vi "yaqc_home.vi"(8 "error in (no error)":errorcluster, 9 "Yaqc Client In":refnum<k38>, 10 "Python Module Path In":path, 11 "Python Session In":refnum<k35>) -> (0 "error out":errorcluster, 1 "Yaqc Client Out":refnum<k38>, 2 "Python Module Path Out":path, 3 "Python Session Out":refnum<k35>)   [LabVIEW 2022 SP3]
doc: "Initiates the homing procedure. The daemon will report as busy during the homing procedure. After the homing procedure is complete, the daemon will return to the current destination."
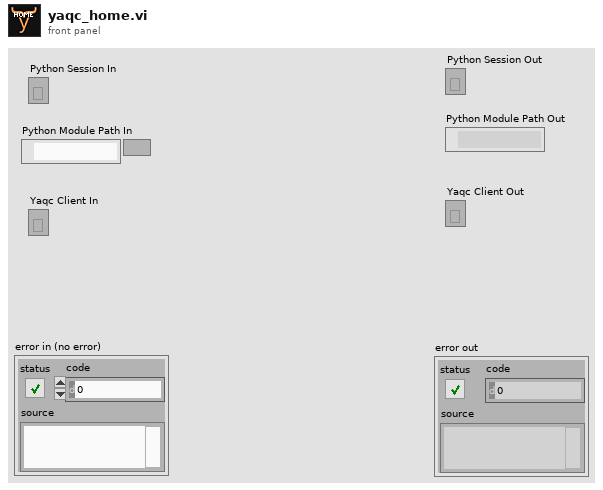
[diagram p1: front panel]
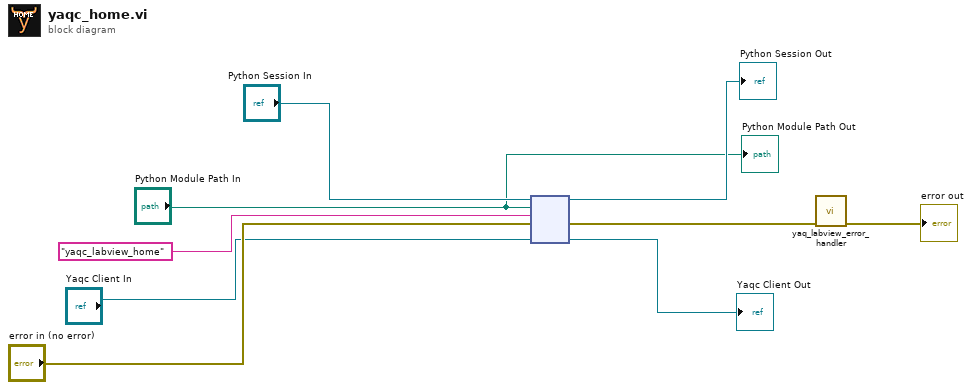
[diagram p0: block diagram]
diagram:
  n1 = node("Python Session In", "Python Module Path In", "yaqc_labview_home" ("function name"), "error in (no error)", "Yaqc Client In") -> (→"Python Session Out":refnum<k35>, w6:errorcluster, →"Yaqc Client Out":refnum<k38>)  [unwired: 2 in, 2 out]
  n2 = call "yaq_labview_error_handler.vi"("error in (no error)"=w6) -> ("error out"=→"error out":errorcluster)  [unwired: 10 in]
  "Python Module Path Out" <- "Python Module Path In"
